vi "Station Shiled Panel.vi"(8 "error in (no error)":errorcluster, 9 "Station Name":string[](array[string])=["Spare", "Spare", "Spare", "Spare", "Spare", "Spare", "Spare", "Spare", "Spare", "Spare", "Spare", "Spare", "Spare", "Spare", "Spare", "Spare"], 10 "Base Path":path=path "D:/Inalfa_Work/Project Program/FTT_Project/TP3_FTT/system", 11 "Shield":u32=1568) -> (0 "error out":errorcluster, 3 "Shield 0ut":u32)   [LabVIEW 2014]
panel:
  in  "Cancel":bool
  in  "Save":bool
  in  "Shield":T1
  # "Station Shield"
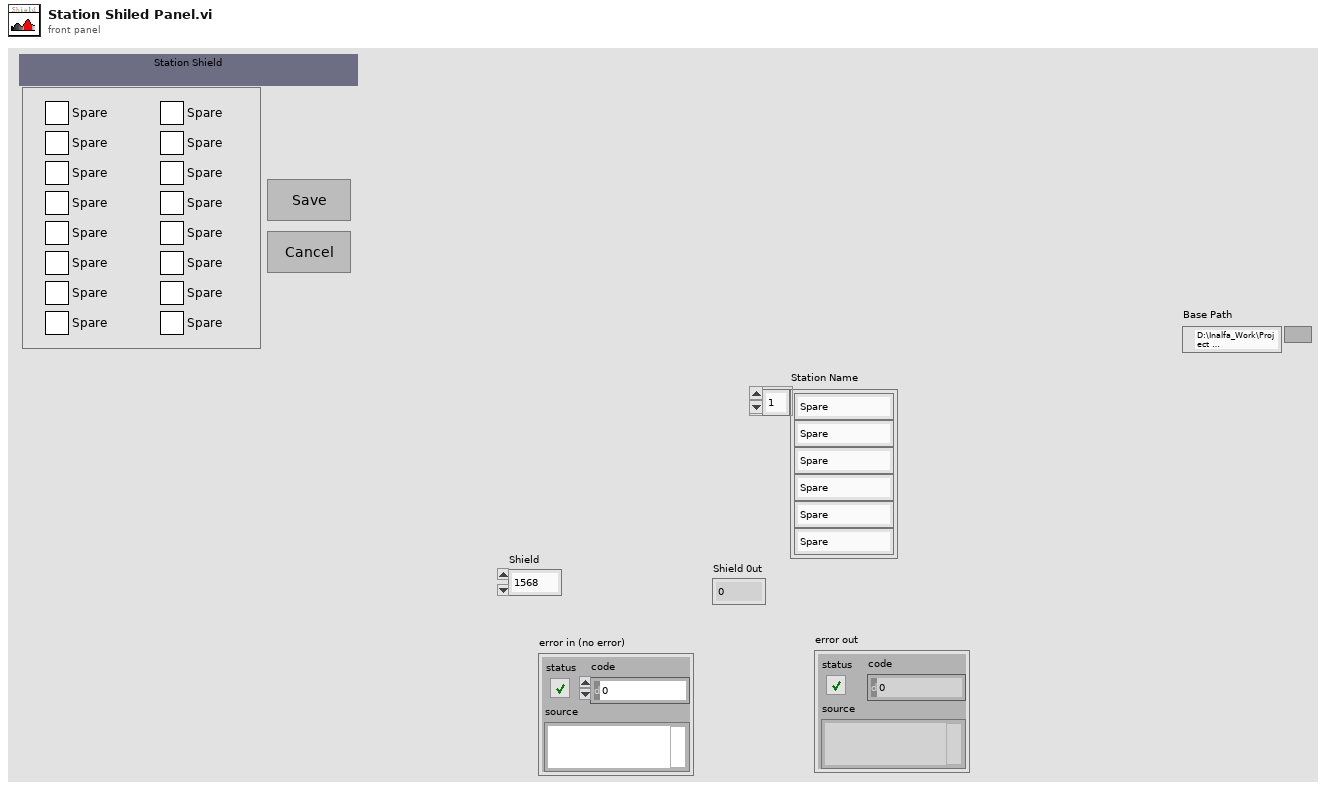
[diagram p1: front panel]
types:
  T1 = cluster{"No.1":bool, "No.2":bool, "No.3":bool, "No.4":bool, "No.5":bool, "No.6":bool, "No.7":bool, "No.8":bool, "No.9":bool, "No.10":bool, "No.10 2":bool, "No.11":bool, "No.12":bool, "No.11 2":bool, "No.12 2":bool, "No.12 3":bool}
  T2 = cluster{"Shield":u32, "Shield":refnum<vi>, "Base Path":path, "Station Name":string[]}
  T3 = cluster{"Boolean array[0]":bool, "Boolean array[1]":bool, "Boolean array[2]":bool, "Boolean array[3]":bool, "Boolean array[4]":bool, "Boolean array[5]":bool, "Boolean array[6]":bool, "Boolean array[7]":bool, "Boolean array[8]":bool, "Boolean array[9]":bool, "Boolean array[10]":bool, "Boolean array[11]":bool, "Boolean array[12]":bool, "Boolean array[13]":bool, "Boolean array[14]":bool, "Boolean array[15]":bool}
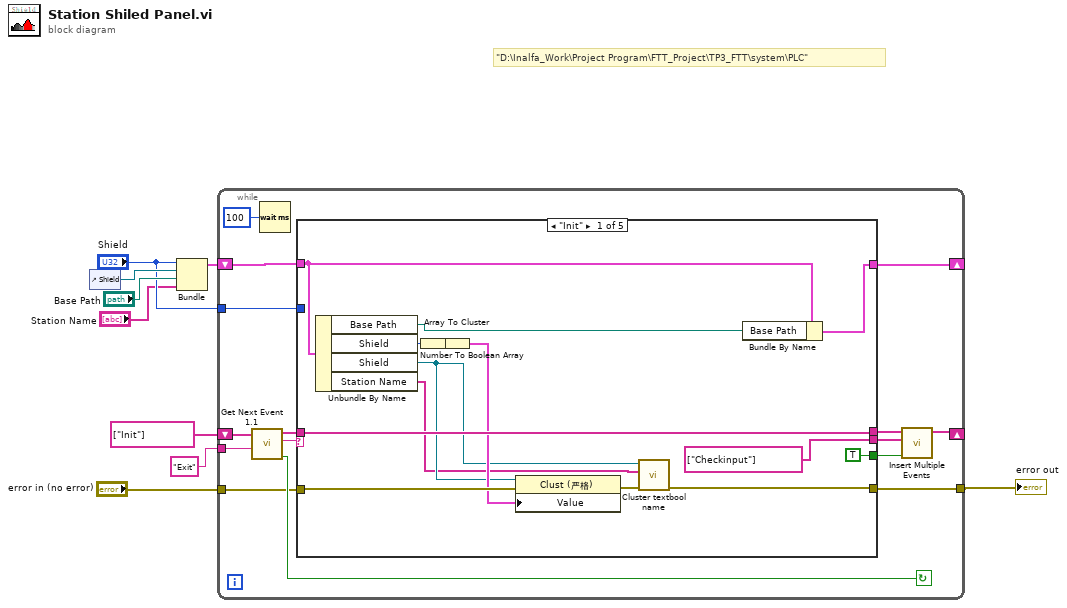
[diagram p0: block diagram]
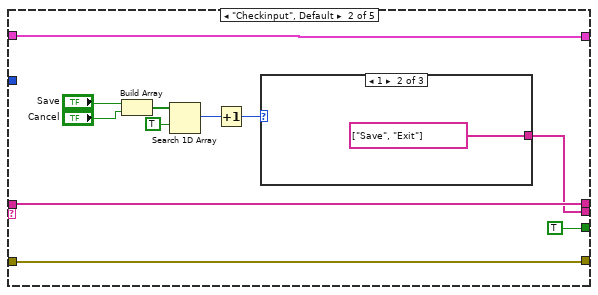
[diagram p2: hidden frame]
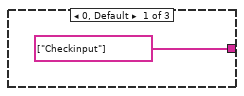
[diagram p3: hidden frame]
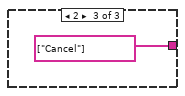
[diagram p4: hidden frame]
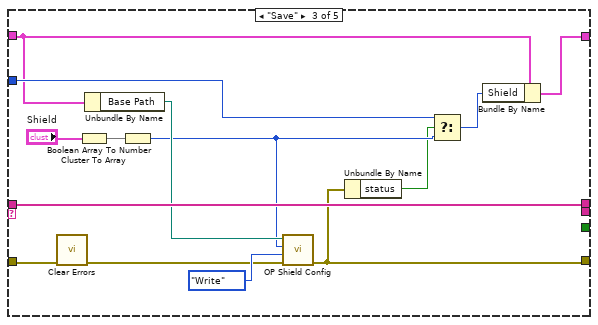
[diagram p5: hidden frame]
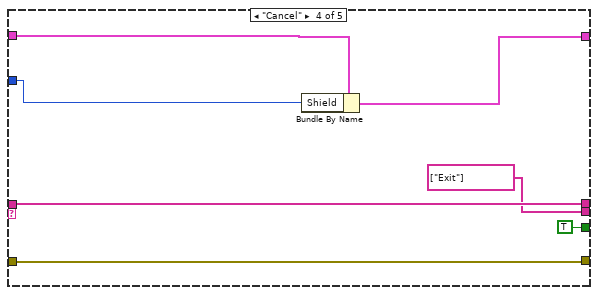
[diagram p6: hidden frame]
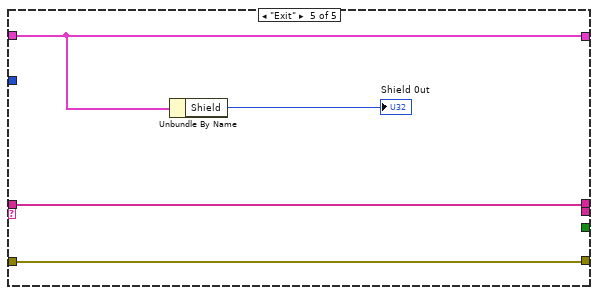
[diagram p7: hidden frame]
diagram:
  # "\"D:\\Inalfa_Work\\Project Program\\FTT_Project\\TP3_FTT\\system\\PLC\""
  n1 = control-ref of="Shield"() -> (w7:refnum<vi>)
  n2 = Bundle("Shield"="Shield", "Shield"=w7, "Base Path"="Base Path", "Station Name"="Station Name") -> (w6:T2)  [unwired: 1 in]
  n3 = while {
    shift-right: [w19] -> _
    shift-left: string[] ["Init"] ("event queue in") -> [w23]
    tunnel: "error in (no error)" -> [w20]
    shift-right: [w14] -> _
    shift-left: w6 -> [w15]
    tunnel: [w13] -> w5
    tunnel: "Exit" -> [w12]
    tunnel: "Shield" -> [w10]
    stop <- w24 continue-if-true
    n4 = call "Get Next Event 1.1.vi"("Exit Event"=w12, "event queue in"=w23) -> ("Condition (Exit:F)"=w24:bool, "next event"=w22:string, "event queue out"=w21:string[])  [unwired: 6 in, 1 out]
    n5 = Wait (ms)(milliseconds to wait=u32 100) -> ()  [unwired: 1 out]
    n6 = case shown="\"Init\"" w22 {
      tunnel: w21 -> [w37 w49 w60 w73 w76]
      tunnel: w20 -> [w33 w39 w54 w72 w77]
      tunnel: [w37 w49 w60 w73 w76] -> w18
      tunnel: [TRUE TRUE _ TRUE _] -> w17
      tunnel: [string[] ["Checkinput"] w41 _ string[] ["Exit"] _] -> w16
      tunnel: w15 -> [w31 w40 w62 w68 w75]
      tunnel: [w30 w40 w61 w67 w75] -> w14
      tunnel: [w26 w39 w56 w72 w77] -> w13
      tunnel: w10 -> [_ _ w64 w69 _]
      frame "Init" {
        n7 = Unbundle By Name(w31) -> ("Base Path"=w25:path, "Shield"=w34:u32, "Shield"=w28:refnum<vi>, "Station Name"=w27:string[])
        n8 = Number To Boolean Array(number=w34) -> (Boolean array=w38:bool[])
        n9 = Array To Cluster(array=w38) -> (cluster=w32:T3)
        n10 = property class="Clust (严格)"(reference=w28, error in=w33, "Value"=w32) -> (error out=w29:errorcluster)  [unwired: 1 out]
        n11 = call "Cluster textbool name.vi"("error in (no error)"=w29, "Station Name"=w27, "Clust Refnum"=w28) -> ("error out"=w26:errorcluster)  [unwired: 8 in]
        n12 = Bundle By Name(cluster=w31, "Base Path"=w25) -> (w30:T2)
      }
      frame "Checkinput", Default {
        n13 = Build Array("Save", "Cancel") -> (w45:bool[])
        n14 = Search 1D Array(1D array=w45, element=TRUE) -> (index of element=w43:i32)  [unwired: 1 in]
        n15 = Increment(x=w43) -> (x+1=w42:i32)
        n16 = case shown="1" w42 {
          tunnel: [string[] ["Checkinput"] string[] ["Save", "Exit"] string[] ["Cancel"]] -> w41
          frame 0, Default {
          }
          frame 1 {
          }
          frame 2 {
          }
        }
      }
      frame "Save" {
        n17 = call <vilib>:"Clear Errors.vi"("error in (no error)"=w54) -> ("error out"=w53:errorcluster)  [unwired: 5 in, 1 out]
        n18 = Cluster To Array(cluster="Shield") -> (array=w65:bool[])
        n19 = Unbundle By Name(w62) -> ("Base Path"=w59:path)
        n20 = Boolean Array To Number(Boolean array=w65) -> (number=w58:u32)
        n21 = call "OP Shield Config.vi"("error in (no error)"=w53, "Enum"=enum16{"init", "Read", "Write"}."Write", "Shield in"=w58, "Path"=w59) -> ("error out"=w56:errorcluster)  [unwired: 4 in, 3 out]
        n22 = Unbundle By Name(w56) -> ("status"=w55:bool)
        n23 = Select(t=w64, s=w55, f=w58) -> (s? t:f=w63:u32)
        n24 = Bundle By Name(cluster=w62, "Shield"=w63) -> (w61:T2)
      }
      frame "Cancel" {
        n25 = Bundle By Name(cluster=w68, "Shield"=w69) -> (w67:T2)
      }
      frame "Exit" {
        n26 = Unbundle By Name(w75) -> ("Shield"=→"Shield 0ut":u32)
      }
    }
    n27 = call "Insert Multiple Events.vi"("Insert all? (T)"=w17, "Events to Insert"=w16, "Event queue in"=w18) -> ("Event queue out"=w19:string[])  [unwired: 4 in]
  }
  "error out" <- w5
